vi "DestroyWindow.vi"(8 "error in (no error)":errorcluster, 11 "Window in":refnum<class "Window.lvclass">) -> (0 "error out":errorcluster, 3 "Window out":refnum<class "Window.lvclass">)   [LabVIEW 2024, in "GLF.lvlib" / "Window.lvclass"]
uses:
  Window.lvclass
  Window.lvclass/Window.ctl
  661d9599-c861-4e81-bf32-b2df16145a3c.vi
  <vilib>/Saukko/LV SDL3/Sources/SDL3/Video/Video.lvlib
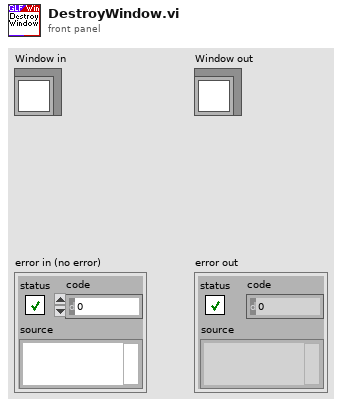
[diagram p1: front panel]
types:
  T1 = typedef "GLF.lvlib/Window.lvclass/DVR--cluster.ctl" = cluster{"SDL_Window *":i64}
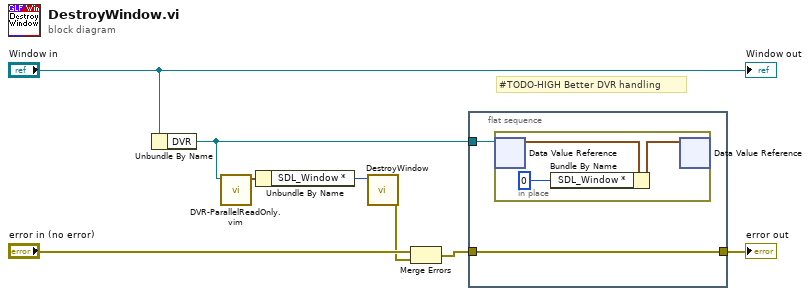
[diagram p0: block diagram]
diagram:
  # "#TODO-HIGH Better DVR handling"
  n1 = Unbundle By Name("Window in") -> ("DVR"=w6:refnum<data-value>)
  n2 = call "DVR-ParallelReadOnly.vim"("DVR"=w6) -> ("Data"=w5:T1)  [unwired: 9 in, 1 out]
  n3 = Unbundle By Name(w5) -> ("SDL_Window *"=w3:i64)
  n4 = call <vilib>:"DestroyWindow.vi"("Window [SDL_Window*]"=w3) -> ("Error Out"=w4:errorcluster)  [unwired: 10 in]
  n5 = Merge Errors("error in (no error)", w4) -> (w2:errorcluster)
  n6 = flat-sequence {
    tunnel: w6 -> [w10]
    tunnel: w2 -> [w9]
    tunnel: [w9] -> w1
    frame #0 {
      n7 = in-place {
        n8 = in-place-dvr #1(w10) -> (w13:T1)  [unwired: 1 out]
        n9 = Bundle By Name(cluster=w13, "SDL_Window *"=i64 0) -> (w12:T1)
        n10 = in-place-dvr #1(w12) -> ()  [unwired: 2 out]
      }
    }
  }
  "error out" <- w1
  "Window out" <- "Window in"
